vi "OEE_SCREEN_1.vi"(8 "error_in":errorcluster, 11 "all_config_info":T2={"main_ini_file"={"SQL Driver"="", "SQL Server"="", "SQL Database"="", "SQL UID"="", "Reference table"="", "Reference history"="", "Archivisation CFG table"="", "Archivisation CFG history"="", "User table"="", "User history"="", "Default reference"="", "Update pulse[ms]"=0, "default language"="", "SCREEN 1 Left"=0, "SCREEN 1 Top"=10, "SCREEN 1 Width"=0, "SCREEN 1 Height"=0, "SCREEN 2 Left"=0, "SCREEN 2 Top"=0, "SCREEN 2 Width"=0, "SCREEN 2 Height"=10}, "SQL Password"="", "queue_refnums"={"MAIN_queue"=refnum, "SCREEN_1_queue"=refnum, "SCREEN_2_queue"=refnum, "PULSE_queue"=refnum, "GRAPH_TOGGLE_queue"=refnum}}) -> (0 "error_out":errorcluster)   [LabVIEW 2019]
uses:
  ini/typedef/OEE_all_config_info.ctl
  ini/typedef/OEE_main_ini_file.ctl
  queues/typedef/OEE_queue_refnums.ctl
  queues/typedef/OEE_MAIN_queue_element.ctl
  MAIN/OEE_MAIN_sequence_state.ctl
  queues/typedef/OEE_SCREEN_1_queue_element.ctl
  OEE_SCREEN_1_sequence_state.ctl
  queues/typedef/OEE_SCREEN_2_queue_element.ctl
  SCREEN_2/OEE_SCREEN_2_sequence_state.ctl
  queues/typedef/OEE_PULSE_queue_element.ctl
  PULSE/OEE_PULSE_sequence_state.ctl
  queues/typedef/OEE_GRAPH_TOGGLE_TIMER_queue_element.ctl
  SCREEN_2/GRAPH_TOGGLE_TIMER/OEE_GRAPH_TOGGLE_TIMER_sequence_state.ctl
  typedef/SCREEN_1.ctl
  typedef/SCREEN_1_recolor_references.ctl
  <vilib>/Utility/miscctls.llb/LVRectTypeDef.ctl
  <vilib>/Utility/error.llb/DialogType.ctl
  _misc/AULocalize/SubVIs/RegisterVI.vi
  _misc/AULocalize/SubVIs/Get Localized Phrase Compact Interface 0D.vi
panel:
  in  "STOP":bool
  out "SCREEN_1":T1={"header_date"="-", "header_time"="-", "header_takt"="-", "header_shift"="-", "OP10_actual"="-", "OP10_rejects"="-", "OP10_quality_yeild"="-", "OP10_pace"="-", "OP20_actual"="-", "OP20_rejects"="-", "OP20_quality_yeild"="-", "OP20_pace"="-", "OP30_actual"="-", "OP30_rejects"="-", "OP30_quality_yeild"="-", "OP30_pace"="-", "OP40_actual"="-", "OP40_rejects"="-", "OP40_quality_yeild"="-", "OP40_pace"="-", "OP50_actual"="-", "OP50_rejects"="-", "OP50_quality_yeild"="-", "OP50_pace"="-", "OP60_actual"="-", "OP60_rejects"="-", "OP60_quality_yeild"="-", "OP60_pace"="-", "OP70_actual"="-", "OP70_rejects"="-", "OP70_quality_yeild"="-", "OP70_pace"="-", "OP80_actual"="-", "OP80_rejects"="-", "OP80_quality_yeild"="-", "OP80_pace"="-", "OP90_actual"="-", "OP90_rejects"="-", "OP90_quality_yeild"="-", "OP90_pace"="-", "OP100_actual"="-", "OP100_rejects"="-", "OP100_quality_yeild"="-", "OP100_pace"="-", "OP110_actual"="-", "OP110_rejects"="-", "OP110_quality_yeild"="-", "OP110_pace"="-", "OP120_actual"="-", "OP120_rejects"="-", "OP120_quality_yeild"="-", "OP120_pace"="-", "OP130_actual"="-", "OP130_rejects"="-", "OP130_quality_yeild"="-", "OP130_pace"="-", "OP10_header"="OP10", "OP20_header"="OP20", "OP30_header"="OP30", "OP40_header"="OP40", "OP50_header"="OP50", "OP60_header"="OP60", "OP70_header"="OP70", "OP80_header"="OP80", "OP90_header"="OP90", "OP100_header"="OP100", "OP110_header"="OP110", "OP120_header"="OP120", "OP130_header"="OP130", "additional_info"="", "bottleneck_OP"="-", "bottleneck_header"="LINE BOTTLENECK", "screen_1_header"="", "actual_header"="", "rejects_header"="", "FTTH_header"="", "pace_header"="", "actual_header"="", "rejects_header"="", "FTTH_header"="", "pace_header"=""}
  # "OP"
  # "OP"
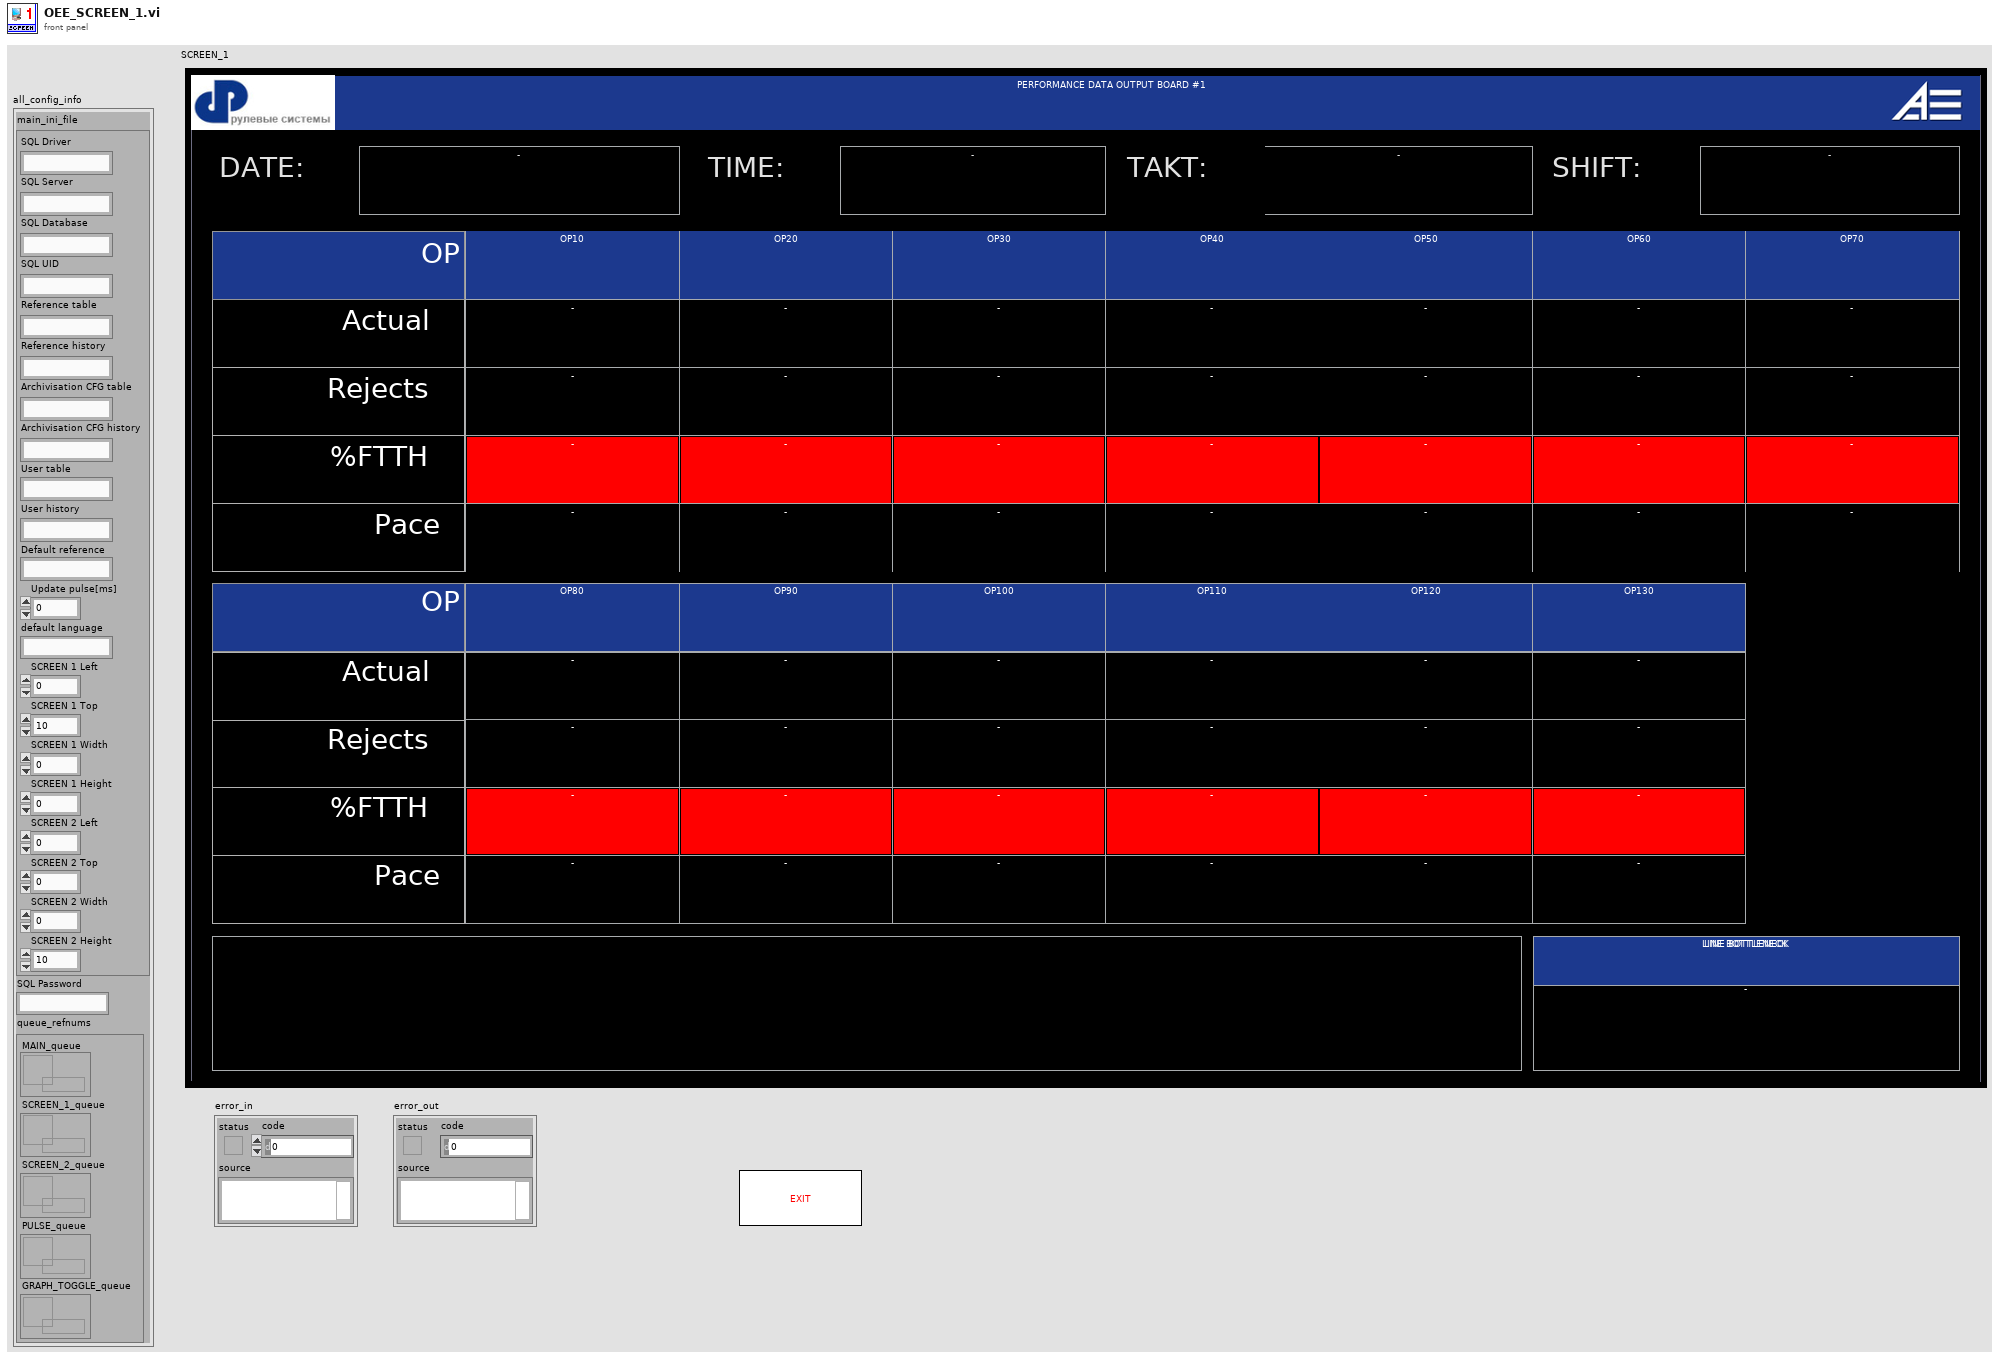
[diagram p1: front panel]
types:
  T1 = typedef "SCREEN_1.ctl" = cluster{"header_date":string, "header_time":string, "header_takt":string, "header_shift":string, "OP10_actual":string, "OP10_rejects":string, "OP10_quality_yeild":string, "OP10_pace":string, "OP20_actual":string, "OP20_rejects":string, "OP20_quality_yeild":string, "OP20_pace":string, "OP30_actual":string, "OP30_rejects":string, "OP30_quality_yeild":string, "OP30_pace":string, "OP40_actual":string, "OP40_rejects":string, "OP40_quality_yeild":string, "OP40_pace":string, "OP50_actual":string, "OP50_rejects":string, "OP50_quality_yeild":string, "OP50_pace":string, "OP60_actual":string, "OP60_rejects":string, "OP60_quality_yeild":string, "OP60_pace":string, "OP70_actual":string, "OP70_rejects":string, "OP70_quality_yeild":string, "OP70_pace":string, "OP80_actual":string, "OP80_rejects":string, "OP80_quality_yeild":string, "OP80_pace":string, "OP90_actual":string, "OP90_rejects":string, "OP90_quality_yeild":string, "OP90_pace":string, "OP100_actual":string, "OP100_rejects":string, "OP100_quality_yeild":string, "OP100_pace":string, "OP110_actual":string, "OP110_rejects":string, "OP110_quality_yeild":string, "OP110_pace":string, "OP120_actual":string, "OP120_rejects":string, "OP120_quality_yeild":string, "OP120_pace":string, "OP130_actual":string, "OP130_rejects":string, "OP130_quality_yeild":string, "OP130_pace":string, "OP10_header":string, "OP20_header":string, "OP30_header":string, "OP40_header":string, "OP50_header":string, "OP60_header":string, "OP70_header":string, "OP80_header":string, "OP90_header":string, "OP100_header":string, "OP110_header":string, "OP120_header":string, "OP130_header":string, "additional_info":string, "bottleneck_OP":string, "bottleneck_header":string, "screen_1_header":string, "actual_header":string, "rejects_header":string, "FTTH_header":string, "pace_header":string, "actual_header":string, "rejects_header":string, "FTTH_header":string, "pace_header":string}
  T2 = typedef "OEE_all_config_info.ctl" = cluster{"main_ini_file":T3, "SQL Password":string, "queue_refnums":T4}
  T3 = typedef "OEE_main_ini_file.ctl" = cluster{"SQL Driver":string, "SQL Server":string, "SQL Database":string, "SQL UID":string, "Reference table":string, "Reference history":string, "Archivisation CFG table":string, "Archivisation CFG history":string, "User table":string, "User history":string, "Default reference":string, "Update pulse[ms]":i32, "default language":string, "SCREEN 1 Left":i16, "SCREEN 1 Top":i16, "SCREEN 1 Width":i16, "SCREEN 1 Height":i16, "SCREEN 2 Left":i16, "SCREEN 2 Top":i16, "SCREEN 2 Width":i16, "SCREEN 2 Height":i16}
  T4 = typedef "OEE_queue_refnums.ctl" = cluster{"MAIN_queue":refnum<queue>, "SCREEN_1_queue":refnum<queue>, "SCREEN_2_queue":refnum<queue>, "PULSE_queue":refnum<queue>, "GRAPH_TOGGLE_queue":refnum<queue>}
  T5 = typedef "LVRectTypeDef.ctl" = cluster{"Left":i16, "Top":i16, "Right":i16, "Bottom":i16}
  T6 = typedef "SCREEN_1_recolor_references.ctl" = cluster{"OP10_quality_yeild":refnum<vi>, "OP20_quality_yeild":refnum<vi>, "OP30_quality_yeild":refnum<vi>, "OP40_quality_yeild":refnum<vi>, "OP50_quality_yeild":refnum<vi>, "OP60_quality_yeild":refnum<vi>, "OP70_quality_yeild":refnum<vi>, "OP80_quality_yeild":refnum<vi>, "OP90_quality_yeild":refnum<vi>, "OP100_quality_yeild":refnum<vi>, "OP110_quality_yeild":refnum<vi>, "OP120_quality_yeild":refnum<vi>, "OP130_quality_yeild":refnum<vi>, "OP10_pace":refnum<vi>, "OP20_pace":refnum<vi>, "OP30_pace":refnum<vi>, "OP40_pace":refnum<vi>, "OP50_pace":refnum<vi>, "OP60_pace":refnum<vi>, "OP70_pace":refnum<vi>, "OP80_pace":refnum<vi>, "OP90_pace":refnum<vi>, "OP100_pace":refnum<vi>, "OP110_pace":refnum<vi>, "OP120_pace":refnum<vi>, "OP130_pace":refnum<vi>}
  T7 = typedef "OEE_SCREEN_1_sequence_state.ctl" = enum16{"initialize", "get_next_state", "update", "show", "hide", "error", "stop"}
  T8 = typedef "OEE_SCREEN_1_queue_element.ctl" = cluster{"state":T7, "variable":variant}
  T9 = typedef "DialogType.ctl" = u16
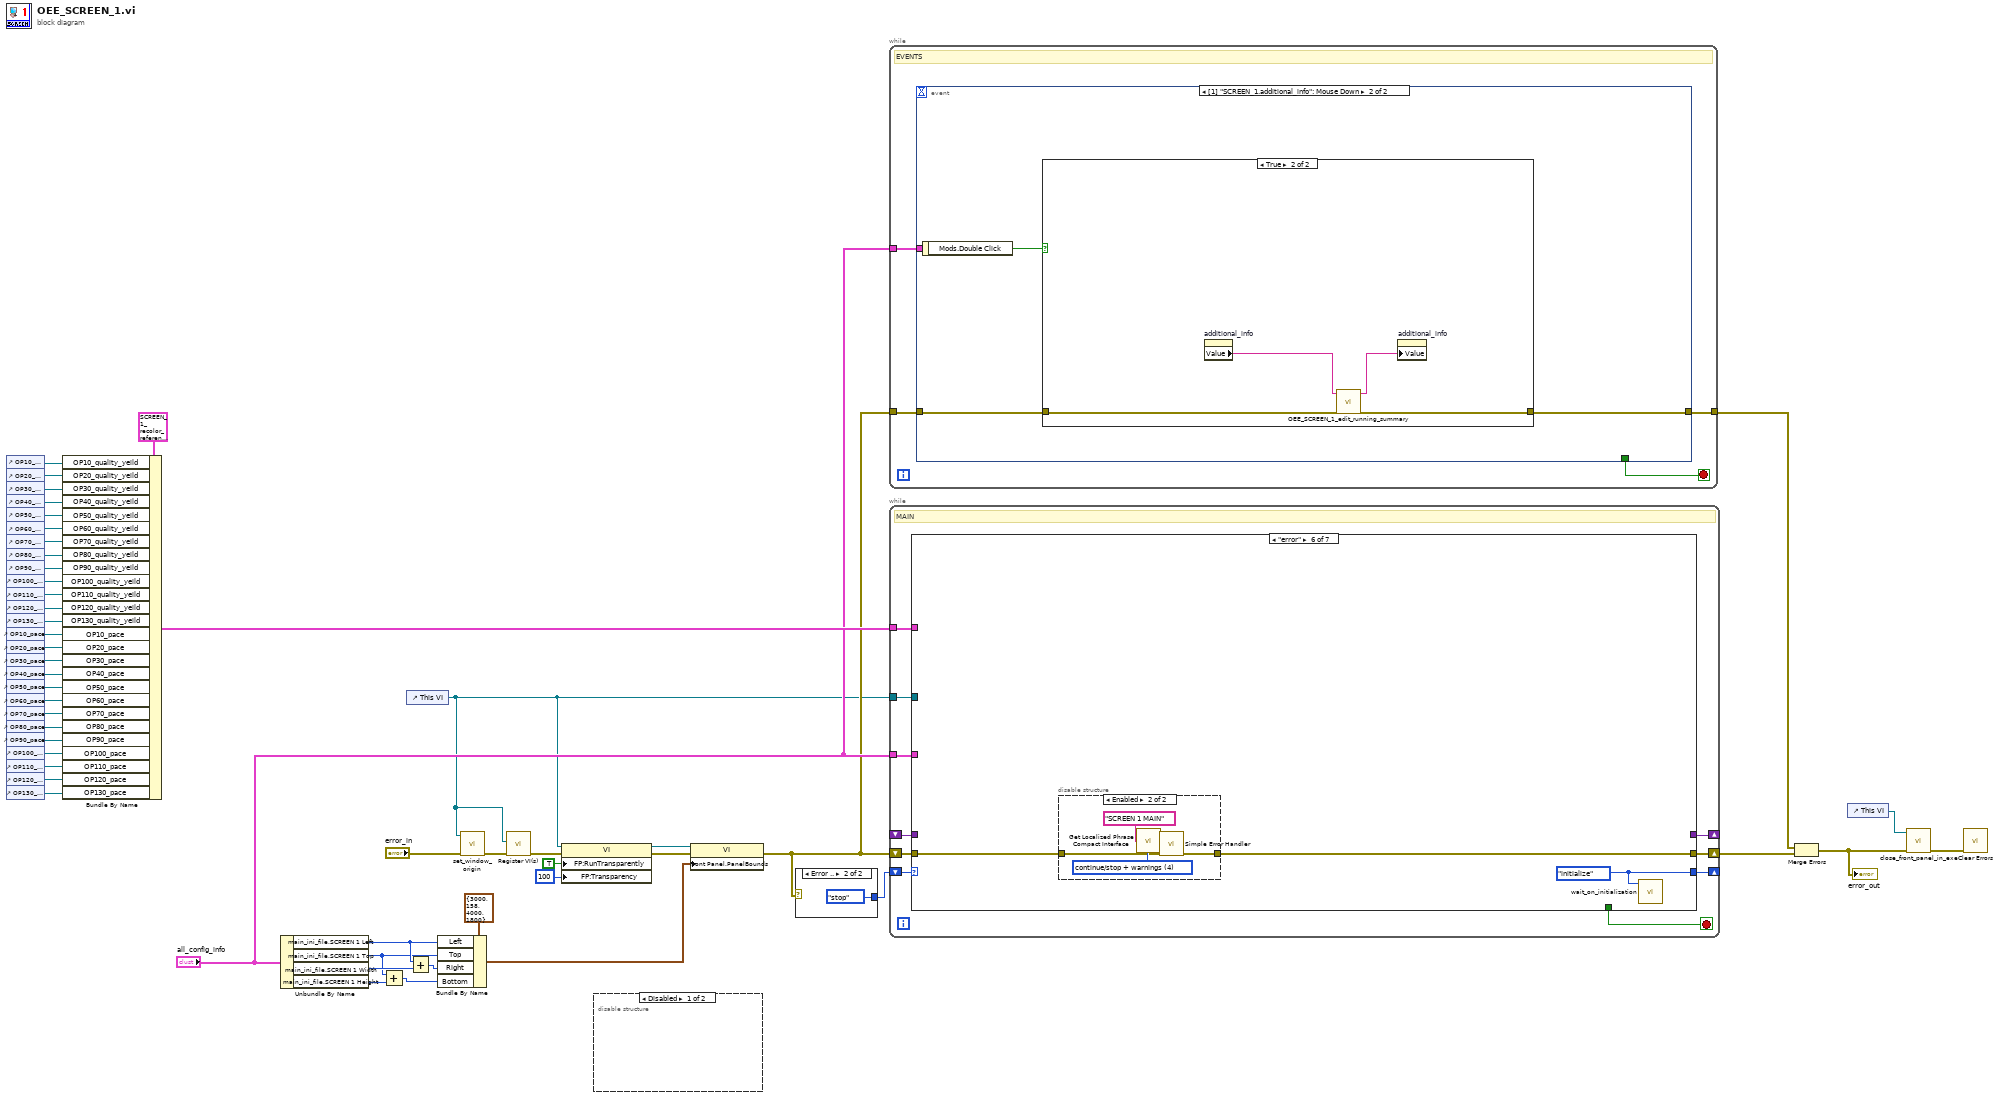
[diagram p0: block diagram]
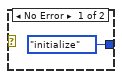
[diagram p3: hidden frame]
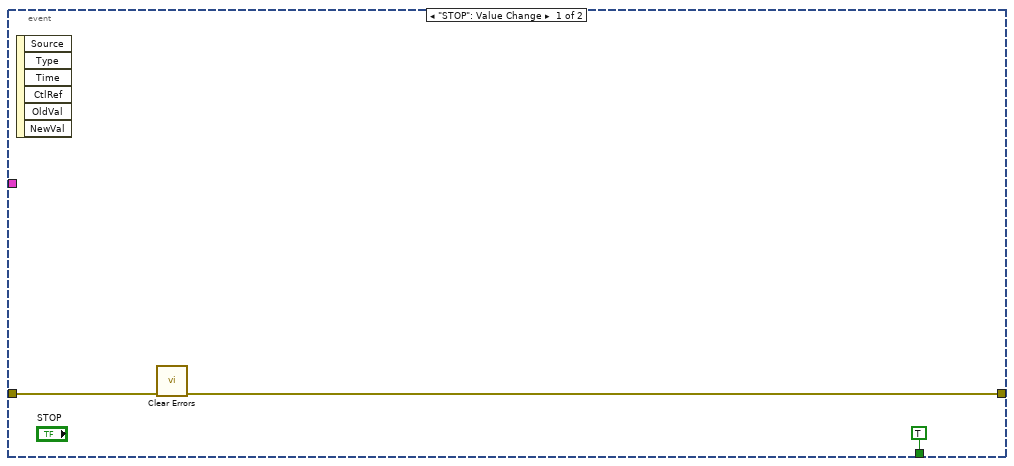
[diagram p4: hidden frame]
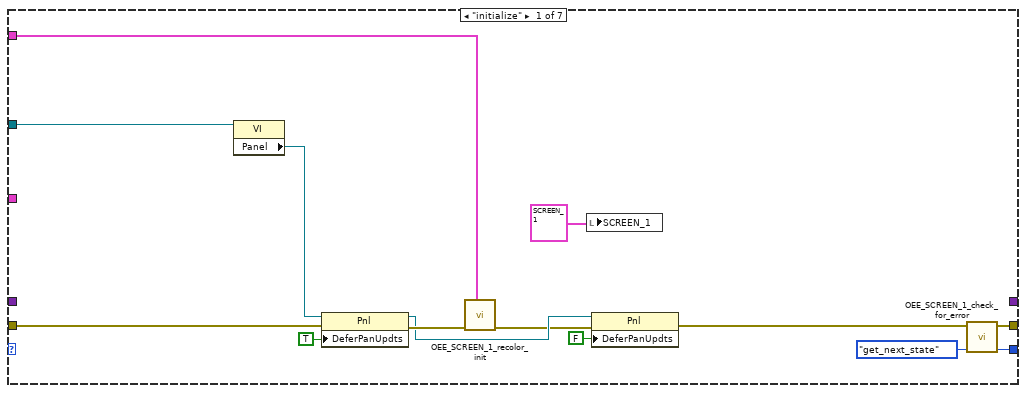
[diagram p6: hidden frame]
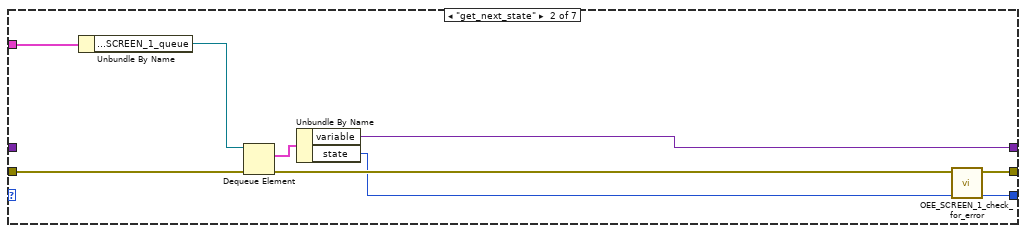
[diagram p7: hidden frame]
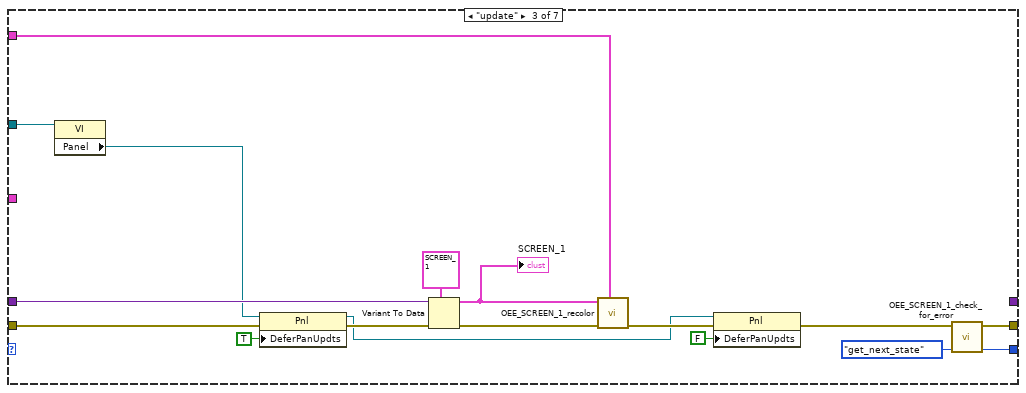
[diagram p8: hidden frame]
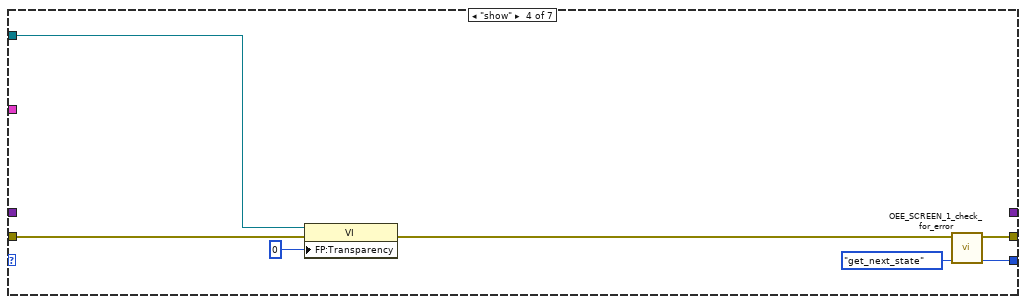
[diagram p9: hidden frame]
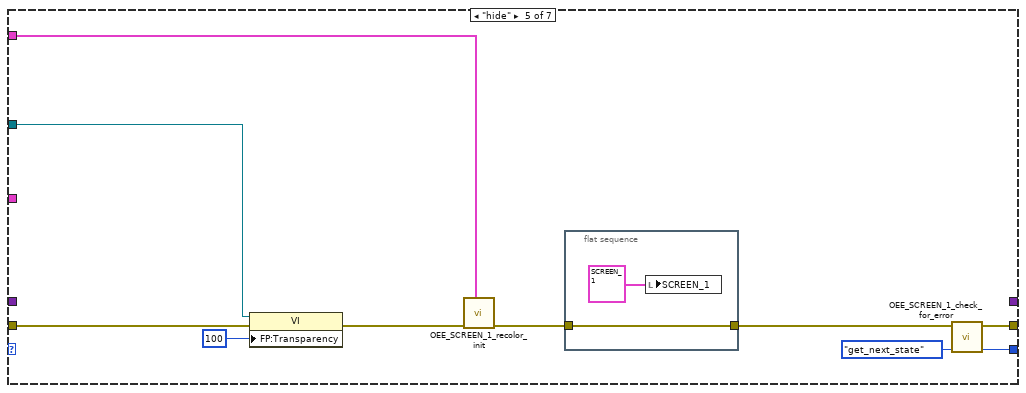
[diagram p10: hidden frame]
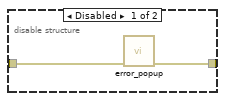
[diagram p11: hidden frame]
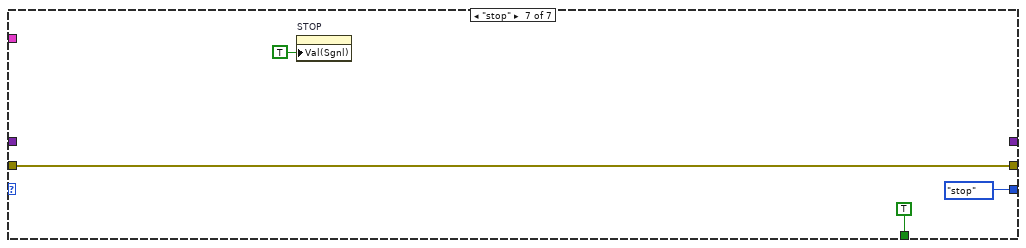
[diagram p12: hidden frame]
diagram:
  n1 = control-ref of="OP10_quality_yeild"() -> (w32:refnum<vi>)
  n2 = control-ref of="OP20_quality_yeild"() -> (w31:refnum<vi>)
  n3 = control-ref of="OP30_quality_yeild"() -> (w30:refnum<vi>)
  n4 = control-ref of="OP40_quality_yeild"() -> (w29:refnum<vi>)
  n5 = control-ref of="OP50_quality_yeild"() -> (w28:refnum<vi>)
  n6 = control-ref of="OP60_quality_yeild"() -> (w27:refnum<vi>)
  n7 = control-ref of="OP70_quality_yeild"() -> (w26:refnum<vi>)
  n8 = control-ref of="OP80_quality_yeild"() -> (w25:refnum<vi>)
  n9 = control-ref of="OP90_quality_yeild"() -> (w24:refnum<vi>)
  n10 = control-ref of="OP100_quality_yeild"() -> (w23:refnum<vi>)
  n11 = control-ref of="OP110_quality_yeild"() -> (w22:refnum<vi>)
  n12 = control-ref of="OP120_quality_yeild"() -> (w21:refnum<vi>)
  n13 = control-ref of="OP130_quality_yeild"() -> (w20:refnum<vi>)
  n14 = control-ref of="OP10_pace"() -> (w19:refnum<vi>)
  n15 = control-ref of="OP20_pace"() -> (w18:refnum<vi>)
  n16 = control-ref of="OP30_pace"() -> (w17:refnum<vi>)
  n17 = control-ref of="OP40_pace"() -> (w16:refnum<vi>)
  n18 = control-ref of="OP50_pace"() -> (w15:refnum<vi>)
  n19 = control-ref of="OP60_pace"() -> (w14:refnum<vi>)
  n20 = control-ref of="OP70_pace"() -> (w13:refnum<vi>)
  n21 = control-ref of="OP80_pace"() -> (w12:refnum<vi>)
  n22 = control-ref of="OP90_pace"() -> (w11:refnum<vi>)
  n23 = control-ref of="OP100_pace"() -> (w10:refnum<vi>)
  n24 = control-ref of="OP110_pace"() -> (w9:refnum<vi>)
  n25 = control-ref of="OP120_pace"() -> (w8:refnum<vi>)
  n26 = control-ref of="OP130_pace"() -> (w7:refnum<vi>)
  n27 = Bundle By Name(cluster=T6 {"OP10_quality_yeild"=refnum, "OP20_quality_yeild"=refnum, "OP30_quality_yeild"=refnum, "OP40_quality_yeild"=refnum, "OP50_quality_yeild"=refnum, "OP60_quality_yeild"=refnum, "OP70_quality_yeild"=refnum, "OP80_quality_yeild"=refnum, "OP90_quality_yeild"=refnum, "OP100_quality_yeild"=refnum, "OP110_quality_yeild"=refnum, "OP120_quality_yeild"=refnum, "OP130_quality_yeild"=refnum, "OP10_pace"=refnum, "OP20_pace"=refnum, "OP30_pace"=refnum, "OP40_pace"=refnum, "OP50_pace"=refnum, "OP60_pace"=refnum, "OP70_pace"=refnum, "OP80_pace"=refnum, "OP90_pace"=refnum, "OP100_pace"=refnum, "OP110_pace"=refnum, "OP120_pace"=refnum, "OP130_pace"=refnum} ("SCREEN_1_recolor_references"), "OP10_quality_yeild"=w32, "OP20_quality_yeild"=w31, "OP30_quality_yeild"=w30, "OP40_quality_yeild"=w29, "OP50_quality_yeild"=w28, "OP60_quality_yeild"=w27, "OP70_quality_yeild"=w26, "OP80_quality_yeild"=w25, "OP90_quality_yeild"=w24, "OP100_quality_yeild"=w23, "OP110_quality_yeild"=w22, "OP120_quality_yeild"=w21, "OP130_quality_yeild"=w20, "OP10_pace"=w19, "OP20_pace"=w18, "OP30_pace"=w17, "OP40_pace"=w16, "OP50_pace"=w15, "OP60_pace"=w14, "OP70_pace"=w13, "OP80_pace"=w12, "OP90_pace"=w11, "OP100_pace"=w10, "OP110_pace"=w9, "OP120_pace"=w8, "OP130_pace"=w7) -> (w49:T6)
  n28 = Unbundle By Name("all_config_info") -> ("main_ini_file.SCREEN 1 Left"=w43:i16, "main_ini_file.SCREEN 1 Top"=w39:i16, "main_ini_file.SCREEN 1 Width"=w42:i16, "main_ini_file.SCREEN 1 Height"=w38:i16)
  n29 = Add(x=w39, y=w38) -> (x+y=w40:i16)
  n30 = control-ref of="This VI"() -> (w1:refnum<vi>)
  n31 = Add(x=w43, y=w42) -> (x+y=w41:i16)
  n32 = Bundle By Name(cluster=T5 {"Left"=3000, "Top"=158, "Right"=4000, "Bottom"=1800} ("Front Panel Window:Panel Bounds"), "Left"=w43, "Top"=w39, "Right"=w41, "Bottom"=w40) -> (w33:T5)
  n33 = call "set_window_origin.vi"("error_in"="error_in", "this_vi_reference"=w1) -> ("error_out"=w3:errorcluster)  [unwired: 9 in]
  n34 = call-poly "Register VI(s).vi"("error in"=w3, "VI Ref"=w1) -> ("error out"=w2:errorcluster)  [unwired: 8 in, 1 out]
  n35 = property class="VI"(reference=w1, error in=w2, "FP:RunTransparently"=TRUE ("Front Panel Window:Run VI Transparently"), "FP:Transparency"=u8 100 ("Front Panel Window:Transparency")) -> (reference out=w34:refnum<vi>, error out=w35:errorcluster)
  n36 = disable-structure shown="Disabled" {
    frame Disabled {
    }
    frame Enabled {
    }
  }
  n37 = property class="VI"(reference=w34, error in=w35, "Front Panel.PanelBounds"=w33) -> (error out=w5:errorcluster)  [unwired: 1 out]
  n38 = case shown="Error .." w5 {
    tunnel: [OEE_SCREEN_1_sequence_state."initialize" ("state") OEE_SCREEN_1_sequence_state."stop" ("state")] -> w45
    frame No Error {
    }
    frame Error {
    }
  }
  n39 = while {
    tunnel: w5 -> [w56]
    tunnel: [w58] -> w46
    tunnel: "all_config_info" -> [w55]
    stop <- w57 stop-if-true
    # "EVENTS"
    n40 = event shown="[1] \"SCREEN_1.additional_info\": Mouse Down" {
      selector: _ -> [_ _]
      dyn-events: _ -> [_ _]
      timeout: _ -> [_ _]
      tunnel: w56 -> [w60 w63]
      tunnel: [w59 w62] -> w58
      tunnel: [TRUE _] -> w57
      tunnel: w55 -> [_ _]
      event "STOP": Value Change {
        n41 = event-data() -> ()  [unwired: 1 in, 6 out]
        n42 = call <vilib>:"Clear Errors.vi"("error in (no error)"=w60) -> ("error out"=w59:errorcluster)  [unwired: 5 in, 1 out]
      }
      event Mouse Down {
        n43 = event-data() -> ("Mods.Double Click"=w64:bool)  [unwired: 1 in]
        n44 = case shown="True" w64 {
          tunnel: w63 -> [w65 w68]
          tunnel: [w65 w69] -> w62
          frame False {
          }
          frame True {
            n45 = property on="additional_info" class="Str"() -> ("Value"=w67:string)  [unwired: 2 in, 2 out]
            n46 = call "OEE_SCREEN_1_edit_running_summary.vi"("error_in"=w68, "running_summary"=w67) -> ("error_out"=w69:errorcluster, "running_summary_updated"=w66:string)  [unwired: 8 in]
            n47 = property on="additional_info" class="Str"("Value"=w66) -> ()  [unwired: 2 in, 2 out]
          }
        }
      }
    }
  }
  n48 = while {
    shift-right: [w76] -> _
    shift-left: w45 -> [w77]
    shift-right: [w75] -> _
    shift-left: _ -> [w74]
    shift-right: [w78] -> w47
    shift-left: w5 -> [w79]
    tunnel: "all_config_info" -> [w72]
    tunnel: w49 -> [w71]
    tunnel: w1 -> [w70]
    stop <- w73 stop-if-true
    # "MAIN"
    n49 = case shown="\"error\"" w77 {
      tunnel: w79 -> [w81 w98 w106 w121 w131 w140 w152]
      tunnel: [w93 w102 w119 w126 w136 w139 w152] -> w78
      tunnel: [w91 w101 w118 w125 w135 w141 OEE_SCREEN_1_sequence_state."stop" ("state")] -> w76
      tunnel: [_ w96 _ _ _ _ _] -> w75
      tunnel: w74 -> [_ _ w116 _ _ _ _]
      tunnel: [_ _ _ _ _ _ TRUE] -> w73
      tunnel: w72 -> [_ w95 _ _ _ _ _]
      tunnel: w71 -> [w90 _ w113 _ w130 _ _]
      tunnel: w70 -> [w82 _ w105 w122 w132 _ _]
      frame "initialize" {
        n50 = property class="VI"(reference=w82) -> ("Panel"=w83:refnum<vi>)  [unwired: 1 in, 2 out]
        n51 = property class="Pnl"(reference=w83, error in=w81, "DeferPanUpdts"=TRUE ("Defer Panel Updates")) -> (reference out=w86:refnum<vi>, error out=w87:errorcluster)
        n52 = call "OEE_SCREEN_1_recolor_init.vi"("SCREEN_1_recolor_references"=w90, "error_in"=w87) -> ("error_out"=w85:errorcluster)  [unwired: 9 in]
        n53 = local write "SCREEN_1"(T1 {"header_date"="-", "header_time"="-", "header_takt"="-", "header_shift"="-", "OP10_actual"="-", "OP10_rejects"="-", "OP10_quality_yeild"="-", "OP10_pace"="-", "OP20_actual"="-", "OP20_rejects"="-", "OP20_quality_yeild"="-", "OP20_pace"="-", "OP30_actual"="-", "OP30_rejects"="-", "OP30_quality_yeild"="-", "OP30_pace"="-", "OP40_actual"="-", "OP40_rejects"="-", "OP40_quality_yeild"="-", "OP40_pace"="-", "OP50_actual"="-", "OP50_rejects"="-", "OP50_quality_yeild"="-", "OP50_pace"="-", "OP60_actual"="-", "OP60_rejects"="-", "OP60_quality_yeild"="-", "OP60_pace"="-", "OP70_actual"="-", "OP70_rejects"="-", "OP70_quality_yeild"="-", "OP70_pace"="-", "OP80_actual"="-", "OP80_rejects"="-", "OP80_quality_yeild"="-", "OP80_pace"="-", "OP90_actual"="-", "OP90_rejects"="-", "OP90_quality_yeild"="-", "OP90_pace"="-", "OP100_actual"="-", "OP100_rejects"="-", "OP100_quality_yeild"="-", "OP100_pace"="-", "OP110_actual"="-", "OP110_rejects"="-", "OP110_quality_yeild"="-", "OP110_pace"="-", "OP120_actual"="-", "OP120_rejects"="-", "OP120_quality_yeild"="-", "OP120_pace"="-", "OP130_actual"="-", "OP130_rejects"="-", "OP130_quality_yeild"="-", "OP130_pace"="-", "OP10_header"="OP10", "OP20_header"="OP20", "OP30_header"="OP30", "OP40_header"="OP40", "OP50_header"="OP50", "OP60_header"="OP60", "OP70_header"="OP70", "OP80_header"="OP80", "OP90_header"="OP90", "OP100_header"="OP100", "OP110_header"="OP110", "OP120_header"="OP120", "OP130_header"="OP130", "additional_info"="", "bottleneck_OP"="-", "bottleneck_header"="", "screen_1_header"="", "actual_header"="", "rejects_header"="", "FTTH_header"="", "pace_header"="", "actual_header"="", "rejects_header"="", "FTTH_header"="", "pace_header"=""} ("SCREEN_1")) -> ()
        n54 = property class="Pnl"(reference=w86, error in=w85, "DeferPanUpdts"=FALSE ("Defer Panel Updates")) -> (error out=w84:errorcluster)  [unwired: 1 out]
        n55 = call "OEE_SCREEN_1_check_for_error.vi"("SCREEN_1_loop_state_in"=OEE_SCREEN_1_sequence_state."get_next_state" ("MAIN_loop_state_in"), "error_in"=w84) -> ("SCREEN_1_loop_state_out"=w91:T7, "error_out"=w93:errorcluster)  [unwired: 8 in]
      }
      frame "get_next_state" {
        n56 = Unbundle By Name(w95) -> ("queue_refnums.SCREEN_1_queue"=w99:refnum<queue>)
        n57 = Dequeue Element(queue=w99, error in (no error)=w98) -> (element=w100:T8, error out=w97:errorcluster)  [unwired: 1 in, 2 out]
        n58 = Unbundle By Name(w100) -> ("variable"=w96:variant, "state"=w94:T7)
        n59 = call "OEE_SCREEN_1_check_for_error.vi"("SCREEN_1_loop_state_in"=w94, "error_in"=w97) -> ("SCREEN_1_loop_state_out"=w101:T7, "error_out"=w102:errorcluster)  [unwired: 8 in]
      }
      frame "update" {
        n60 = property class="VI"(reference=w105) -> ("Panel"=w104:refnum<vi>)  [unwired: 1 in, 2 out]
        n61 = property class="Pnl"(reference=w104, error in=w106, "DeferPanUpdts"=TRUE ("Defer Panel Updates")) -> (reference out=w107:refnum<vi>, error out=w111:errorcluster)
        n62 = Variant To Data(error in=w111, type=T1 {"header_date"="-", "header_time"="-", "header_takt"="-", "header_shift"="-", "OP10_actual"="-", "OP10_rejects"="-", "OP10_quality_yeild"="-", "OP10_pace"="-", "OP20_actual"="-", "OP20_rejects"="-", "OP20_quality_yeild"="-", "OP20_pace"="-", "OP30_actual"="-", "OP30_rejects"="-", "OP30_quality_yeild"="-", "OP30_pace"="-", "OP40_actual"="-", "OP40_rejects"="-", "OP40_quality_yeild"="-", "OP40_pace"="-", "OP50_actual"="-", "OP50_rejects"="-", "OP50_quality_yeild"="-", "OP50_pace"="-", "OP60_actual"="-", "OP60_rejects"="-", "OP60_quality_yeild"="-", "OP60_pace"="-", "OP70_actual"="-", "OP70_rejects"="-", "OP70_quality_yeild"="-", "OP70_pace"="-", "OP80_actual"="-", "OP80_rejects"="-", "OP80_quality_yeild"="-", "OP80_pace"="-", "OP90_actual"="-", "OP90_rejects"="-", "OP90_quality_yeild"="-", "OP90_pace"="-", "OP100_actual"="-", "OP100_rejects"="-", "OP100_quality_yeild"="-", "OP100_pace"="-", "OP110_actual"="-", "OP110_rejects"="-", "OP110_quality_yeild"="-", "OP110_pace"="-", "OP120_actual"="-", "OP120_rejects"="-", "OP120_quality_yeild"="-", "OP120_pace"="-", "OP130_actual"="-", "OP130_rejects"="-", "OP130_quality_yeild"="-", "OP130_pace"="-", "OP10_header"="OP10", "OP20_header"="OP20", "OP30_header"="OP30", "OP40_header"="OP40", "OP50_header"="OP50", "OP60_header"="OP60", "OP70_header"="OP70", "OP80_header"="OP80", "OP90_header"="OP90", "OP100_header"="OP100", "OP110_header"="OP110", "OP120_header"="OP120", "OP130_header"="OP130", "additional_info"="", "bottleneck_OP"="-", "bottleneck_header"="", "screen_1_header"="", "actual_header"="", "rejects_header"="", "FTTH_header"="", "pace_header"="", "actual_header"="", "rejects_header"="", "FTTH_header"="", "pace_header"=""} ("SCREEN_1"), Variant=w116) -> (data=w114:T1, error out=w115:errorcluster)
        "SCREEN_1" <- w114
        n63 = call "OEE_SCREEN_1_recolor.vi"("SCREEN_1_recolor_references"=w113, "error_in"=w115, "SCREEN_1"=w114) -> ("error_out"=w109:errorcluster)  [unwired: 8 in]
        n64 = property class="Pnl"(reference=w107, error in=w109, "DeferPanUpdts"=FALSE ("Defer Panel Updates")) -> (error out=w108:errorcluster)  [unwired: 1 out]
        n65 = call "OEE_SCREEN_1_check_for_error.vi"("SCREEN_1_loop_state_in"=OEE_SCREEN_1_sequence_state."get_next_state", "error_in"=w108) -> ("SCREEN_1_loop_state_out"=w118:T7, "error_out"=w119:errorcluster)  [unwired: 8 in]
      }
      frame "show" {
        n66 = property class="VI"(reference=w122, error in=w121, "FP:Transparency"=u8 0 ("Front Panel Window:Transparency")) -> (error out=w120:errorcluster)  [unwired: 1 out]
        n67 = call "OEE_SCREEN_1_check_for_error.vi"("SCREEN_1_loop_state_in"=OEE_SCREEN_1_sequence_state."get_next_state", "error_in"=w120) -> ("SCREEN_1_loop_state_out"=w125:T7, "error_out"=w126:errorcluster)  [unwired: 8 in]
      }
      frame "hide" {
        n68 = property class="VI"(reference=w132, error in=w131, "FP:Transparency"=u8 100 ("Front Panel Window:Transparency")) -> (error out=w127:errorcluster)  [unwired: 1 out]
        n69 = call "OEE_SCREEN_1_recolor_init.vi"("SCREEN_1_recolor_references"=w130, "error_in"=w127) -> ("error_out"=w129:errorcluster)  [unwired: 9 in]
        n70 = flat-sequence {
          tunnel: w129 -> [w138]
          tunnel: [w138] -> w128
          frame #0 {
            n71 = local write "SCREEN_1"(T1 {"header_date"="-", "header_time"="-", "header_takt"="-", "header_shift"="-", "OP10_actual"="-", "OP10_rejects"="-", "OP10_quality_yeild"="-", "OP10_pace"="-", "OP20_actual"="-", "OP20_rejects"="-", "OP20_quality_yeild"="-", "OP20_pace"="-", "OP30_actual"="-", "OP30_rejects"="-", "OP30_quality_yeild"="-", "OP30_pace"="-", "OP40_actual"="-", "OP40_rejects"="-", "OP40_quality_yeild"="-", "OP40_pace"="-", "OP50_actual"="-", "OP50_rejects"="-", "OP50_quality_yeild"="-", "OP50_pace"="-", "OP60_actual"="-", "OP60_rejects"="-", "OP60_quality_yeild"="-", "OP60_pace"="-", "OP70_actual"="-", "OP70_rejects"="-", "OP70_quality_yeild"="-", "OP70_pace"="-", "OP80_actual"="-", "OP80_rejects"="-", "OP80_quality_yeild"="-", "OP80_pace"="-", "OP90_actual"="-", "OP90_rejects"="-", "OP90_quality_yeild"="-", "OP90_pace"="-", "OP100_actual"="-", "OP100_rejects"="-", "OP100_quality_yeild"="-", "OP100_pace"="-", "OP110_actual"="-", "OP110_rejects"="-", "OP110_quality_yeild"="-", "OP110_pace"="-", "OP120_actual"="-", "OP120_rejects"="-", "OP120_quality_yeild"="-", "OP120_pace"="-", "OP130_actual"="-", "OP130_rejects"="-", "OP130_quality_yeild"="-", "OP130_pace"="-", "OP10_header"="OP10", "OP20_header"="OP20", "OP30_header"="OP30", "OP40_header"="OP40", "OP50_header"="OP50", "OP60_header"="OP60", "OP70_header"="OP70", "OP80_header"="OP80", "OP90_header"="OP90", "OP100_header"="OP100", "OP110_header"="OP110", "OP120_header"="OP120", "OP130_header"="OP130", "additional_info"="", "bottleneck_OP"="-", "bottleneck_header"="", "screen_1_header"="", "actual_header"="", "rejects_header"="", "FTTH_header"="", "pace_header"="", "actual_header"="", "rejects_header"="", "FTTH_header"="", "pace_header"=""} ("SCREEN_1")) -> ()
          }
        }
        n72 = call "OEE_SCREEN_1_check_for_error.vi"("SCREEN_1_loop_state_in"=OEE_SCREEN_1_sequence_state."get_next_state", "error_in"=w128) -> ("SCREEN_1_loop_state_out"=w135:T7, "error_out"=w136:errorcluster)  [unwired: 8 in]
      }
      frame "error" {
        w141 = OEE_SCREEN_1_sequence_state."initialize" ("state")
        n73 = disable-structure shown="Enabled" {
          disable-tunnel: w140 -> [w143 w145]
          disable-tunnel: [w142 w148] -> w139
          frame Disabled {
            n74 = call "error_popup.vi"("error_in"=w143) -> ("error_out"=w142:errorcluster)  [unwired: 10 in]
          }
          frame Enabled {
            w146 = T9 4 items=["no dialog", "OK message", "continue or stop message", "OK message + warnings", "continue/stop + warnings"] ("type of dialog (OK msg:1)")
            n75 = call-poly "Get Localized Phrase Compact Interface.vi"("Key"="SCREEN 1 MAIN" ("error source (\" \")")) -> ("Translated Phrase"=w144:string)
            n76 = call <vilib>:"Simple Error Handler.vi"("error source (\" \")"=w144, "type of dialog (OK msg:1)"=w146, "error in (no error)"=w145) -> ("error out"=w148:errorcluster)  [unwired: 2 in, 4 out]
          }
        }
        n77 = call "wait_on_initialization.vi"("state"=w141) -> ()  [unwired: 11 in]
      }
      frame "stop" {
        n78 = property on="STOP" class="Bool (strict)"("Val(Sgnl)"=TRUE ("Value (Signaling)")) -> ()  [unwired: 2 in, 2 out]
      }
    }
  }
  n79 = Merge Errors(w46, w47) -> (w6:errorcluster)
  "error_out" <- w6
  n80 = control-ref of="This VI"() -> (w52:refnum<vi>)
  n81 = call "close_front_panel_in_exe.vi"("error_in"=w6, "vi_reference_in"=w52) -> ("error_out"=w51:errorcluster)  [unwired: 9 in]
  n82 = call <vilib>:"Clear Errors.vi"("error in (no error)"=w51) -> ()  [unwired: 5 in, 2 out]
